vi "Save_File_Sample_Setup.vi"(8 "Error In":errorcluster, 9 "input cluster":T1={"L16 Linear Actuator"="", "XE 1000 Pump"="", "Camera1"="", "Camera2"="", "Camera1_IMG"=refnum, "Camera2_IMG"=refnum, "Img_Capt"=FALSE, "Actuator"=FALSE, "Pump"=FALSE, "Cam 1"=FALSE, "Cam 2"=FALSE, "Empty_Refill"=FALSE, "Crop"=FALSE, "Light intensity"=100, "Exposure Time"=1000.0, "Sample Name"="Test Sample", "Operator"="MRJ", "Calibration 1"=path "C:/Users/au540322/Desktop/IHS_Project/images/Debris/Debris_0/Debris_0_2019_06_01-23-32-49-686.PNG", "Calibration 2"=path "C:/Users/au540322/Desktop/IHS_Project/images/Debris/Debris_0/Debris_0_2019_06_01-23-32-49-686.PNG", "Framerate"=1, "Timeout Sample"=50, "Collection date"="MRJ", "Sample size threshold"=1, "Empty start"=1, "Command"="MRJ", "Calibration Image 1"=refnum, "Calibration Image 2"=refnum, "Original Image 1"=refnum, "Original Image 2"=refnum, "Processing Image 1"=refnum, "Processing Image 2"=refnum, "Object Image 1"=refnum, "Object Image 2"=refnum, "Station"="", "Species Name"="", "Other Notes"="", "Aperture"=enum."Item 0", "Image Process Queue Size"=500, "Image Save Queue Size"=500, "Overload threshold"=500, "Max Framerate"=100, "Blue Plane Image"=refnum, "Subtract Image"=refnum, "Binary Image 1"=refnum, "ROI mask allocation"=refnum, "Rectangle 1"={"Left"=0, "Top"=0, "Right"=0, "Bottom"=0, "Rotation"=0.0}, "Rectangle 2"={"Left"=0, "Top"=0, "Right"=0, "Bottom"=0, "Rotation"=0.0}, "Binary Image 2"=refnum, "Detection Region %"=0.0, "Cam 1 queue"=refnum, "Cam 2 queue"=refnum, "Detect image 1"=refnum, "Detect image 2"=refnum, "Detect 1"=path "C:/Users/au540322/Desktop/IHS_Project/images/Debris/Debris_0/Debris_0_2019_06_01-23-32-49-686.PNG", "Detect 2"=path "C:/Users/au540322/Desktop/IHS_Project/images/Debris/Debris_0/Debris_0_2019_06_01-23-32-49-686.PNG", "Max large object threshold"=0, "Open(T)/Close(F)"=FALSE, "Cam 1 - save queue"=refnum, "Cam 2 - save queue"=refnum, "Img_Capt Begin"=FALSE} {"Rectangle 2"."Rotation" format="%.2f"; "Rectangle 2"."Left" scale=0.0..1024.0; "Rectangle 2"."Right" scale=0.0..1024.0; "Rectangle 1"."Rotation" format="%.2f"; "Rectangle 1"."Left" scale=0.0..1024.0; "Rectangle 1"."Right" scale=0.0..1024.0; "Max Framerate" min=1; "Overload threshold" min=1; "Image Save Queue Size" min=1; "Image Process Queue Size" min=1; "Empty start" min=1; "Sample size threshold" min=1; "Framerate" min=1; "Light intensity" scale=0.0..100.0}, 11 "Sample Subfolder Name":string) -> (0 "Error Out":errorcluster)   [LabVIEW 2019]
doc: "Save a file containing current sample setup information:\n\nCamera settings\n- Exposure Time [µs]\n- Light Intensity [%]\n- Sample Frequency [FPS]\n\nOperator\n- Name\n- Sample Notes/Description\n\nDate\n- DDMMYYYY"
uses:
  controls/Data.ctl
  <vilib>/userdefined/High Color/IMAQdx.ctl
  <vilib>/vision/Image Controls.llb/IMAQ Image.ctl
  <vilib>/Utility/config.llb/Write Key (String).vi
  <vilib>/Utility/config.llb/NI_LVConfig.lvlib
panel:
  out "?":errorcluster
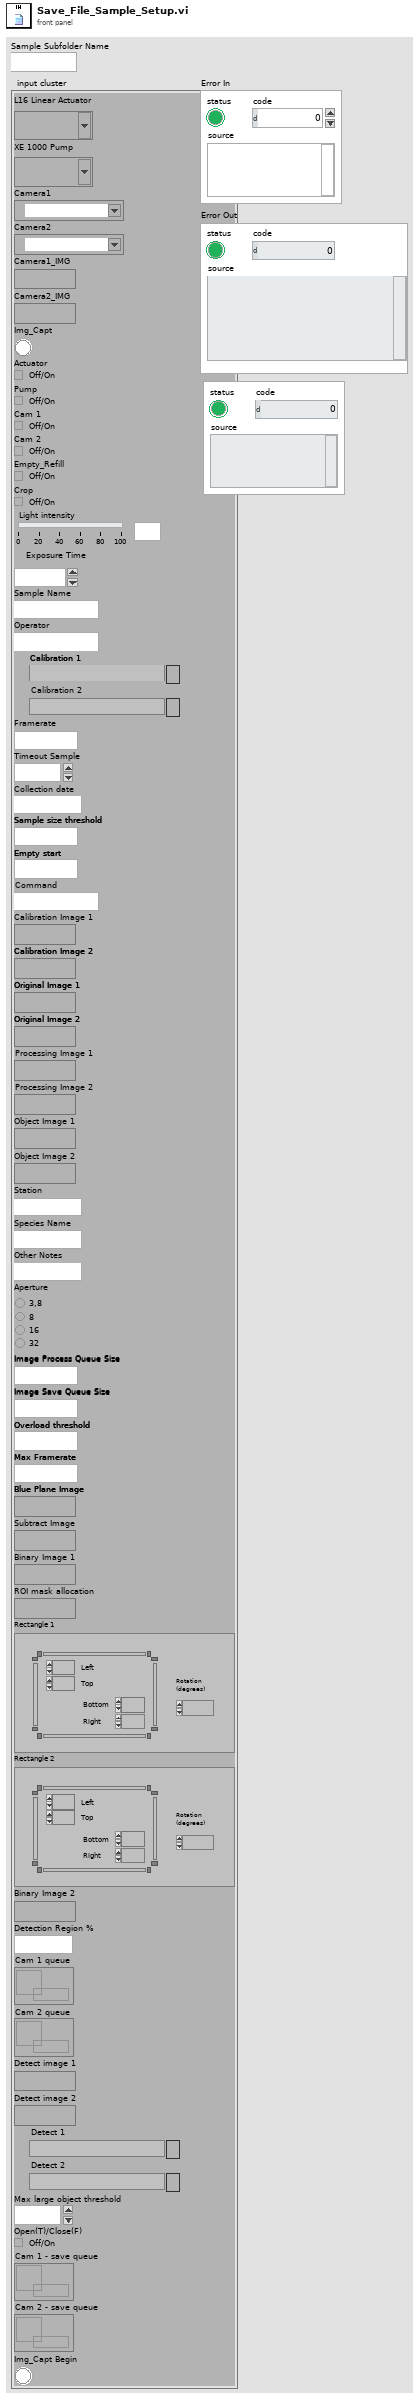
[diagram p1: front panel]
types:
  T1 = typedef "Data.ctl" = cluster{"L16 Linear Actuator":refnum<visa-resource-name>, "XE 1000 Pump":refnum<visa-resource-name>, "Camera1":T2, "Camera2":T2, "Camera1_IMG":T3, "Camera2_IMG":T3, "Img_Capt":bool, "Actuator":bool, "Pump":bool, "Cam 1":bool, "Cam 2":bool, "Empty_Refill":bool, "Crop":bool, "Light intensity":i32, "Exposure Time":dbl, "Sample Name":string, "Operator":string, "Calibration 1":path, "Calibration 2":path, "Framerate":i32, "Timeout Sample":i32, "Collection date":string, "Sample size threshold":i32, "Empty start":u32, "Command":string, "Calibration Image 1":T3, "Calibration Image 2":T3, "Original Image 1":T3, "Original Image 2":T3, "Processing Image 1":T3, "Processing Image 2":T3, "Object Image 1":T3, "Object Image 2":T3, "Station":string, "Species Name":string, "Other Notes":string, "Aperture":enum32{"Item 0", "Item 1", "Item 2", "Item 3"}, "Image Process Queue Size":i32, "Image Save Queue Size":i32, "Overload threshold":i32, "Max Framerate":i32, "Blue Plane Image":T3, "Subtract Image":T3, "Binary Image 1":T3, "ROI mask allocation":T3, "Rectangle 1":T4, "Rectangle 2":T4, "Binary Image 2":T3, "Detection Region %":dbl, "Cam 1 queue":refnum<queue>, "Cam 2 queue":refnum<queue>, "Detect image 1":T3, "Detect image 2":T3, "Detect 1":path, "Detect 2":path, "Max large object threshold":i32, "Open(T)/Close(F)":bool, "Cam 1 - save queue":refnum<queue>, "Cam 2 - save queue":refnum<queue>, "Img_Capt Begin":bool}
  T2 = typedef "IMAQdx.ctl" = refnum<k21>
  T3 = typedef "IMAQ Image.ctl" = refnum<image>
  T4 = typedef "IMAQ Rectangle" = cluster{"Left":i32, "Top":i32, "Right":i32, "Bottom":i32, "Rotation":dbl}
  T5 = typedef "NI_LVConfig.lvlib/Config Data RefNum.ctl" = refnum<k1>
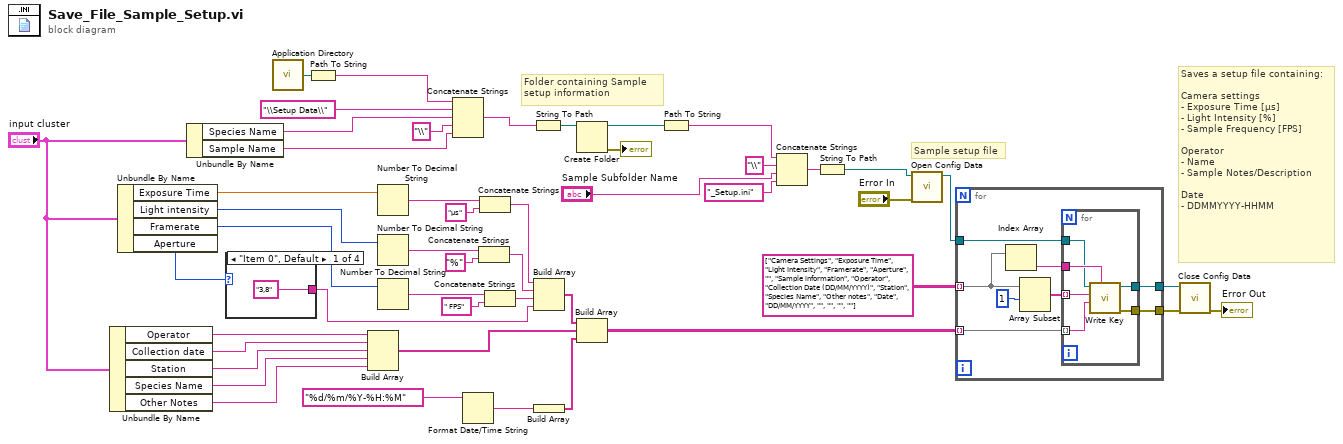
[diagram p0: block diagram]
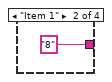
[diagram p2: hidden frame]
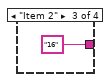
[diagram p3: hidden frame]
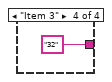
[diagram p4: hidden frame]
diagram:
  # "Saves a setup file containing:\n\nCamera settings\n- Exposure Time [µs]\n- Light Intensity [%]\n- Sample Frequency [FPS]\n\nOperator\n- Name\n- Sample Notes/Description\n\nDate\n- DDMMYYYY-HHMM"
  # "Sample setup file"
  # "Folder containing Sample \nsetup information"
  n1 = Unbundle By Name("input cluster") -> ("Operator"=w8:string, "Collection date"=w7:string, "Station"=w6:string, "Species Name"=w5:string, "Other Notes"=w4:string)
  n2 = Unbundle By Name("input cluster") -> ("Exposure Time"=w27:dbl, "Light intensity"=w26:i32, "Framerate"=w15:i32, "Aperture"=w3:enum32{"Item 0", "Item 1", "Item 2", "Item 3"})
  n3 = Unbundle By Name("input cluster") -> ("Species Name"=w13:string, "Sample Name"=w11:string)
  n4 = case shown="\"Item 0\", Default" w3 {
    tunnel: ["3,8" "8" "16" "32"] -> w2
    frame "Item 0", Default {
    }
    frame "Item 1" {
    }
    frame "Item 2" {
    }
    frame "Item 3" {
    }
  }
  n5 = call <vilib>:"Application Directory.vi"() -> ("Application Directory"=w37:path)
  n6 = Path To String(path=w37) -> (string=w35:string)
  n7 = Build Array(w8, w7, w6, w5, w4) -> (w14:string[])
  n8 = Number To Decimal String(number=w27) -> (decimal integer string=w21:string)  [unwired: 1 in]
  n9 = Number To Decimal String(number=w26) -> (decimal integer string=w23:string)  [unwired: 1 in]
  n10 = Number To Decimal String(number=w15) -> (decimal integer string=w18:string)  [unwired: 1 in]
  n11 = Concatenate Strings(w35, "\\Setup Data\\" ("string"), w13, "\\" ("string"), w11) -> (w10:string)
  n12 = Format Date/Time String(time format string (%c)="%d/%m/%Y-%H:%M") -> (date/time string=w38:string)  [unwired: 2 in]
  n13 = Concatenate Strings(w23, "%" ("string")) -> (w22:string)
  n14 = Concatenate Strings(w21, "µs" ("string")) -> (w19:string)
  n15 = Concatenate Strings(w18, " FPS" ("string")) -> (w17:string)
  n16 = String To Path(string=w10) -> (path=w34:path)
  n17 = Build Array(w19, w22, w17, w2) -> (w48:string[])
  n18 = Build Array(w38) -> (w39:string[])
  n19 = Create Folder(path (use dialog)=w34) -> (created path=w32:path, error out=→"?":errorcluster)  [unwired: 2 in, 1 out]
  n20 = Build Array(w48, w14, w39) -> (w47:string[][])
  n21 = Path To String(path=w32) -> (string=w31:string)
  n22 = Concatenate Strings(w31, "\\" ("string"), "Sample Subfolder Name", "_Setup.ini" ("string")) -> (w41:string)
  n23 = String To Path(string=w41) -> (path=w43:path)
  n24 = call <vilib>:"Open Config Data.vi"("error in (no error)"="Error In", "configuration file path"=w43) -> ("refnum"=w44:T5)  [unwired: 7 in, 2 out]
  n25 = for {
    tunnel: string[][] [["Camera Settings", "Exposure Time", "Light Intensity", "Framerate", "Aperture", ""], ["Sample information", "Operator", "Collection Date (DD/MM/YYYY)", "Station", "Species Name", "Other notes"], ["Date", "DD/MM/YYYY", "", "", "", ""]] ("appended array") -> [w59] mode=indexing
    tunnel: w47 -> [w57] mode=indexing
    tunnel: [w55] -> w46
    tunnel: [w54] -> w45
    tunnel: w44 -> [w53]
    n26 = Index Array(array=w59) -> (element=w58:string)  [unwired: 1 in]
    n27 = Array Subset(array=w59, index=1) -> (w56:string[])  [unwired: 1 in]
    n28 = for {
      tunnel: w58 -> [w66]
      tunnel: w57 -> [w65] mode=indexing
      tunnel: w56 -> [w64] mode=indexing
      tunnel: [w63] -> w55
      tunnel: [w62] -> w54
      tunnel: w53 -> [w61]
      n29 = call-poly <vilib>:"Write Key.vi"("section"=w66, "value"=w65, "key"=w64, "refnum"=w61) -> ("error out"=w62:errorcluster, "refnum out"=w63:T5)  [unwired: 5 in, 1 out]
    }
  }
  n30 = call <vilib>:"Close Config Data.vi"("error in (no error)"=w45, "refnum"=w46) -> ("error out"=→"Error Out":errorcluster)  [unwired: 8 in, 1 out]
